vi "Execute Key Query.vi"(4 "Section queries":refnum<class "CConfig Query.lvclass">[](array[class]), 5 "Key name":string, 6 "Key queries":refnum<class "CConfig Query.lvclass">[](array[class]), 7 "Section name":string, 8 "error in (no error)":errorcluster, 9 "Use Key Regex? [F]":bool, 10 "Use Section Regex? [F]":bool, 11 "Carya Config in":refnum<class "Carya Config.lvclass">) -> (0 "error out":errorcluster, 2 "Results":string[][](array[string]), 3 "Carya Config out":refnum<class "Carya Config.lvclass">)   [LabVIEW 2013, in "Carya Config.lvclass"]
doc: "Copyright 2018, Carya Automatisering, Wiebe Walstra."
uses:
  Carya Config.lvclass
  CConfig Object/CConfig Query.lvclass
  CConfig Object/Step In Query/Step In Query.lvclass
  CConfig Object/Composite Query/Composite Query.lvclass
  CConfig Object/Loop Query/Match Query/Match Query.lvclass
  CConfig Object/Loop Query/All Query/All Query.lvclass
  CConfig Object/Loop Query/All Type Query/All Type Query.lvclass
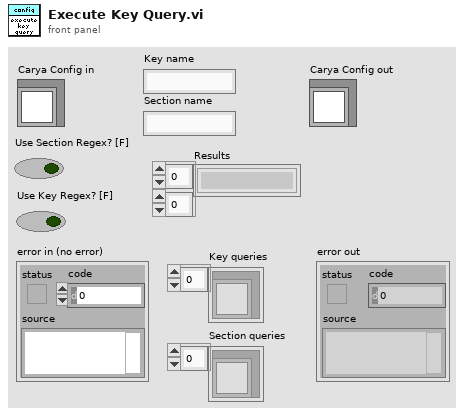
[diagram p1: front panel]
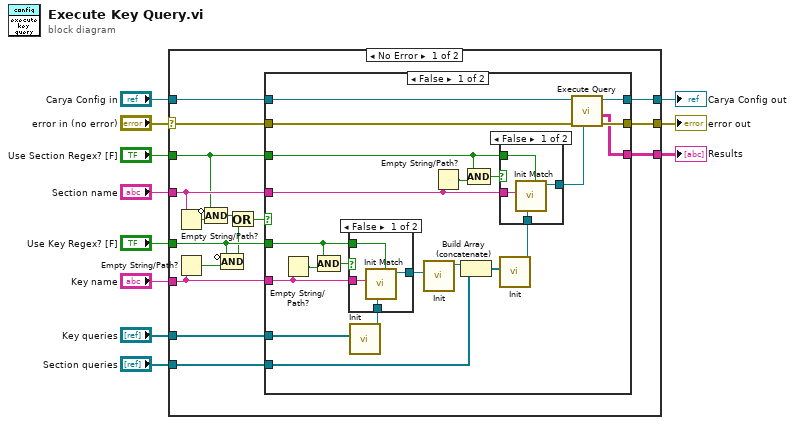
[diagram p0: block diagram]
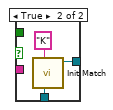
[diagram p2: hidden frame]
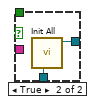
[diagram p3: hidden frame]
diagram:
  n1 = case shown="No Error" "error in (no error)" {
    selector: "error in (no error)" -> [w27 w65]
    tunnel: [w16 w65] -> w8
    tunnel: [w15 w64] -> w9
    tunnel: "Carya Config in" -> [w17 w64]
    tunnel: "Section name" -> [w26 _]
    tunnel: "Use Section Regex? [F]" -> [w23 _]
    tunnel: "Key name" -> [w20 _]
    tunnel: "Use Key Regex? [F]" -> [w19 _]
    tunnel: "Key queries" -> [w14 _]
    tunnel: "Section queries" -> [w13 _]
    tunnel: [w12 _] -> w1
    frame No Error {
      n2 = Empty String/Path?(string/path=w26) -> (empty?=w25:bool)
      n3 = Empty String/Path?(string/path=w20) -> (empty?=w22:bool)
      n4 = Compound Arithmetic op=AND(invert w23, w25) -> (w21:bool)
      n5 = Compound Arithmetic op=AND(invert w19, w22) -> (w18:bool)
      n6 = Or(x=w21, y=w18) -> (x .or. y?=w24:bool)
      n7 = case shown="False" w24 {
        tunnel: w17 -> [w45 w63]
        tunnel: w26 -> [w40 _]
        tunnel: w23 -> [w41 _]
        tunnel: w20 -> [w35 _]
        tunnel: [w44 w63] -> w15
        tunnel: w19 -> [w34 _]
        tunnel: w27 -> [w37 w62]
        tunnel: [w48 w62] -> w16
        tunnel: w14 -> [w30 _]
        tunnel: w13 -> [w29 _]
        tunnel: [w28 _] -> w12
        frame False {
          n8 = Empty String/Path?(string/path=w35) -> (empty?=w36:bool)
          n9 = Compound Arithmetic op=AND(w34, w36) -> (w32:bool)
          n10 = call "Init.vi"("Queries"=w30) -> ("Step In Query out"=w31:refnum<class "CConfig Query.lvclass">)  [unwired: 9 in, 1 out]
          n11 = case shown="False" w32 {
            tunnel: w34 -> [w51 _]
            tunnel: w35 -> [w52 _]
            tunnel: w31 -> [w50 w55]
            tunnel: [w49 w54] -> w33
            frame False {
              n12 = call "Init Match.vi"("Regex [F]"=w51, "Found"=w50, "Data"=w52) -> ("Find First Query out"=w49:refnum<class "Loop Query.lvclass">)  [unwired: 7 in, 1 out]
            }
            frame True {
              n13 = call "Init Match.vi"("Found"=w55, "Data [name]"="K") -> ("Find First Query out"=w54:refnum<class "Loop Query.lvclass">)  [unwired: 8 in, 1 out]
            }
          }
          n14 = call "Init.vi"("Config Query"=w33) -> ("Step In Query out"=w46:refnum<class "Step In Query.lvclass">)  [unwired: 9 in, 1 out]
          n15 = Empty String/Path?(string/path=w40) -> (empty?=w42:bool)
          n16 = Build Array (concatenate)(w46, w29) -> (w47:refnum<class "CConfig Query.lvclass">[])
          n17 = Compound Arithmetic op=AND(w41, w42) -> (w43:bool)
          n18 = call "Init.vi"("Queries"=w47) -> ("Step In Query out"=w38:refnum<class "CConfig Query.lvclass">)  [unwired: 9 in, 1 out]
          n19 = case shown="False" w43 {
            tunnel: w41 -> [w58 _]
            tunnel: w40 -> [w59 _]
            tunnel: w38 -> [w57 w61]
            tunnel: [w56 w60] -> w39
            frame False {
              n20 = call "Init Match.vi"("Regex [F]"=w58, "Found"=w57, "Data"=w59) -> ("Find First Query out"=w56:refnum<class "Loop Query.lvclass">)  [unwired: 7 in, 1 out]
            }
            frame True {
              n21 = call "Init All.vi"("Found"=w61) -> ("Find First Query out"=w60:refnum<class "All Query.lvclass">)  [unwired: 9 in, 1 out]
            }
          }
          n22 = call-dynamic "Execute Query.vi"("Config Query in"=w39, "error in (no error)"=w37, "Carya Config in"=w45) -> ("error out"=w48:errorcluster, "Results"=w28:string[][], "Carya Config out"=w44:refnum<class "Carya Config.lvclass">)  [unwired: 4 in, 2 out]
        }
        frame True {
        }
      }
    }
    frame Error {
    }
  }
  "error out" <- w8
  "Carya Config out" <- w9
  "Results" <- w1
